vi "WILT Get Agilent Channels.vi"(10 "all rows":string[][](array[string]), 11 "Agilent Channel":string) -> (3 "Agilent Control":T1[](array[typedef]))   [LabVIEW 2016]
uses:
  Type Definitions/WILT Agilent Channel Definition.ctl
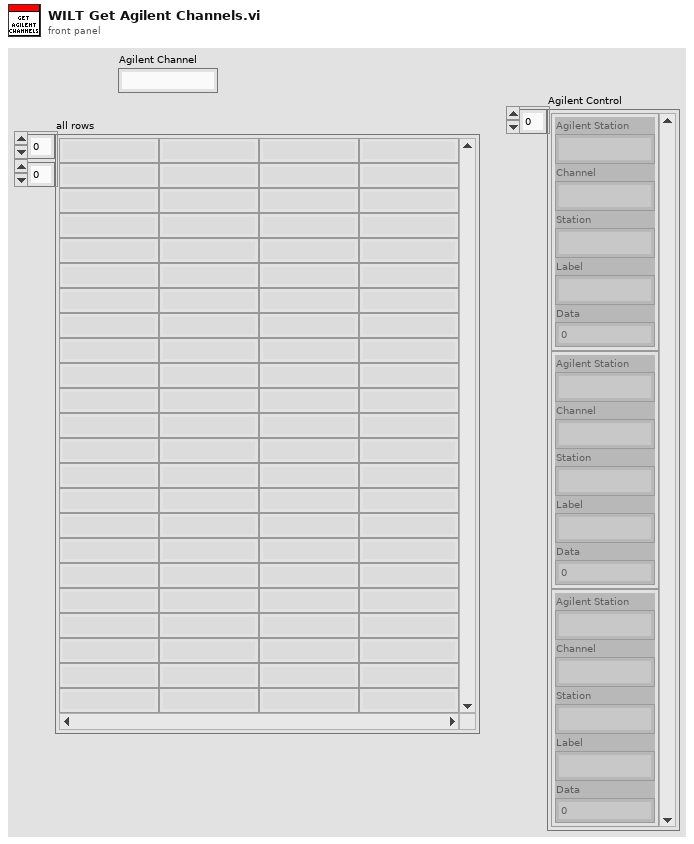
[diagram p1: front panel]
types:
  T1 = typedef "WILT Agilent Channel Definition.ctl" = cluster{"Channel":string, "Station":string, "Label":string, "Agilent Station":string, "Data":dbl}
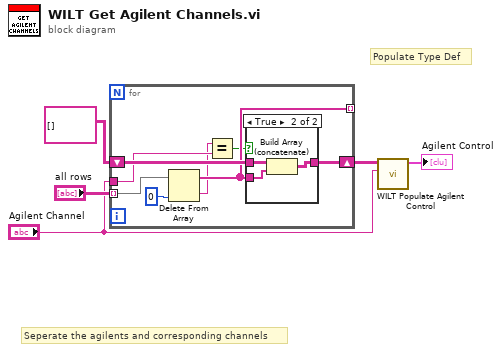
[diagram p0: block diagram]
diagram:
  # "Populate Type Def"
  # "Seperate the agilents and corresponding channels"
  n1 = for {
    tunnel: "all rows" -> [w13] mode=indexing
    shift-right: [w11] -> w3
    shift-left: string[][] [] -> [w10]
    tunnel: "Agilent Channel" -> [w9]
    tunnel: [w8] -> _ mode=indexing
    n2 = Delete From Array(array=w13, index=0) -> (deleted portion=w7:string, array with subset deleted=w8:string[])  [unwired: 1 in]
    n3 = Equal?(x=w7, y=w9) -> (x = y?=w6:bool)
    n4 = case shown="True" w6 {
      tunnel: [w14 w17] -> w11
      tunnel: w10 -> [w14 w16]
      tunnel: w8 -> [_ w15]
      frame False {
      }
      frame True {
        n5 = Build Array (concatenate)(w16, w15) -> (w17:string[][])
      }
    }
  }
  n6 = call "WILT Populate Agilent Control.vi"("Channel"="Agilent Channel", "Agilent1 Channels"=w3) -> ("Agilent Control"=→"Agilent Control":T1[])  [unwired: 9 in]
